vi "GUI_HTU_Camera_presets.vi"() -> ()   [LabVIEW 2013]
uses:
  Shared/GUI_Template/GUI_master/tcp_new_data_event.ctl
  Shared/GUI_Template/GUI_master/tcp new data cluster.ctl
panel:
  in  "OapIn2AA":dbl=0.01
  in  "OapIn1AA":dbl=0.001
  in  "expanderIn2AA":dbl=0.0001
  in  "compInAA":dbl=0.001
  in  "BeamlineOutAA":dbl=0.0001
  in  "BeamlineInAA":dbl=0.0001
  in  "tubeInAA":dbl=0.0001
  in  "DMSurfaceAA":dbl=0.01
  in  "BcaveInAA":dbl=0.0001
  in  "group4":bool caption="Blank Button"
  in  "group3":bool caption="Blank Button"
  in  "amp2inputAA 2":dbl=0.001
  in  "amp3inputAA 2":dbl=0.001
  in  "amp4inputAA 2":dbl=0.001
  in  "amp4outputAA 2":dbl=0.001
  in  "BcaveInAA 2":dbl=0.002
  in  "DMSurfaceAA 2":dbl=0.8
  in  "tubeInAA 2":dbl=0.02
  in  "BeamlineInAA 2":dbl=0.01
  in  "BeamlineOutAA 2":dbl=0.08
  in  "compInAA 2":dbl=0.07
  in  "expanderIn2AA 2":dbl=0.005
  in  "OapIn1AA 2":dbl=0.2
  in  "OapIn2AA 2":dbl=0.8
  in  "amp4outputAA":dbl=0.9
  in  "amp4inputAA":dbl=0.7
  in  "amp3inputAA":dbl=0.5
  in  "group2":bool caption="Blank Button"
  in  "amp2inputAA":dbl=0.002
  in  "exposure::18":dbl caption="TubeIn" min=50.0 max=500000.0
  in  "exposure::17":dbl caption="OapIn2" min=0.0001 max=1.0
  in  "exposure::16":dbl caption="OapIn1" min=0.0001 max=1.0
  in  "exposure::15":dbl caption="ModeImager" min=2e-05 max=1.0
  in  "exposure::14":dbl caption="GratingMode" min=1e-05 max=1.0
  in  "exposure::13":dbl caption="GhostPulsed" min=0.0 max=1.0
  in  "exposure::12":dbl caption="ExpanderIn2" min=3e-05 max=1.0
  in  "exposure::11":dbl caption="ExpanderIn1Pulsed" min=1e-06 max=1.0
  in  "exposure::10":dbl caption="ExapnderIn1" min=3e-05 max=1.0
  in  "exposure::9":dbl caption="DMSurface" min=20.0 max=1000000.0
  in  "exposure::8":dbl caption="compIn" min=2e-05 max=4.0
  in  "exposure::7":dbl caption="beamlineOUt" min=0.0001 max=1.0
  in  "exposure::6":dbl caption="beamlineIn" min=0.0001 max=1.0
  in  "exposure::5":dbl caption="bcavein" min=10.0 max=1000000.0
  in  "exposure::4":dbl caption="amp4Outpur" min=-25.0 max=25.0
  in  "exposure::3":dbl caption="Amp4input" min=0.0001 max=1.0
  in  "exposure::2":dbl caption="amp3input" min=0.0001 max=1.0
  in  "ms exposure":dbl=0.001
  in  "group1":bool caption="Blank Button"
  in  "GUIdevice 18":string="UC_TubeIn"
  in  "GUIdevice 17":string="UC_OAPin2"
  in  "GUIdevice 16":string="UC_OAPin1"
  in  "GUIdevice 15":string="UC_ModeImager"
  in  "GUIdevice 14":string="UC_GratingMode"
  in  "GUIdevice 13":string="UC_Ghost_Pulsed"
  in  "GUIdevice 12":string="UC_ExpanderIn2"
  in  "GUIdevice 11":string="UC_ExpanderIn1_Pulsed"
  in  "GUIdevice 10":string="UC_ExpanderIn1"
  in  "GUIdevice 9":string="UC_DMSurface"
  in  "GUIdevice 8":string="UC_CompIn"
  in  "exposure::1":dbl caption="amp2Input" min=0.0001 max=1.0
  in  "GUIdevice 6":string="UC_Beamline_In"
  in  "GUIdevice 5":string="UC_BCaveIn"
  out "error IO 2":errorcluster
  out "tcp data event":T1
  in  "UDP error message":string
  in  "GUIdevice 7":string="UC_Beamline_Out"
  in  "GUIdevice 2":string="UC_Amp3_IR_input"
  in  "GUIdevice 4":string="UC_Amp4_output"
  in  "GUIdevice 1":string="UC_Amp2_IR_input"
  in  "GUIdevice 3":string="UC_Amp4_IR_input"
  in  "stop":bool
  # "Camera exposure controls"
  # "Direct control"
  # "Energy"
  # "CAP"
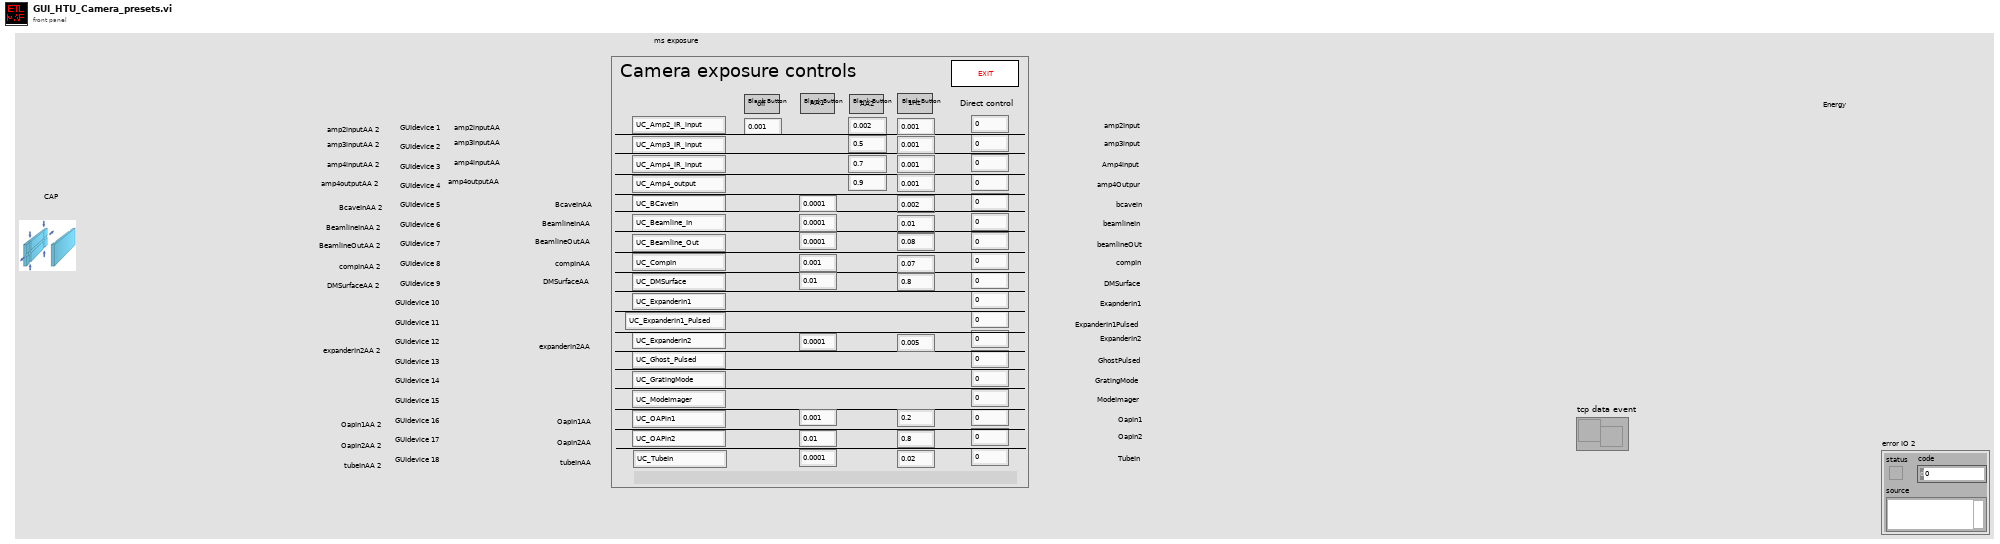
[diagram p1: front panel]
types:
  T1 = typedef "tcp_new_data_event.ctl" = refnum<user-event>
  T2 = typedef "tcp new data cluster.ctl" = cluster{"EventEnum":enum16{"new data", "connection status update"}, "Device name":string}
  T3 = enum32{"invalid app kind", "Development System", "Run Time System", "Student Edition", "Embedded LabVIEW", "Evaluation", "Custom"}
  T4 = enum32{"Invalid", "Standard", "Closed", "Hidden", "Minimized", "Maximized"}
  T5 = cluster{"Core":cluster{"Current VI Reference":refnum<vi>, "Close Panel on Exit?":bool}, "Heater timing offset":dbl, "Discharge timing offset":dbl, "Jet trigger":bool, "Tik1":u32, "Tik2":u32, "Fire Continues Allowed":bool, "Jet enable":bool, "Wedge enable":bool, "Phosphor enable":bool, "last chart update tck":i32}
  T6 = cluster{"Current VI Reference":refnum<vi>, "Close Panel on Exit?":bool}
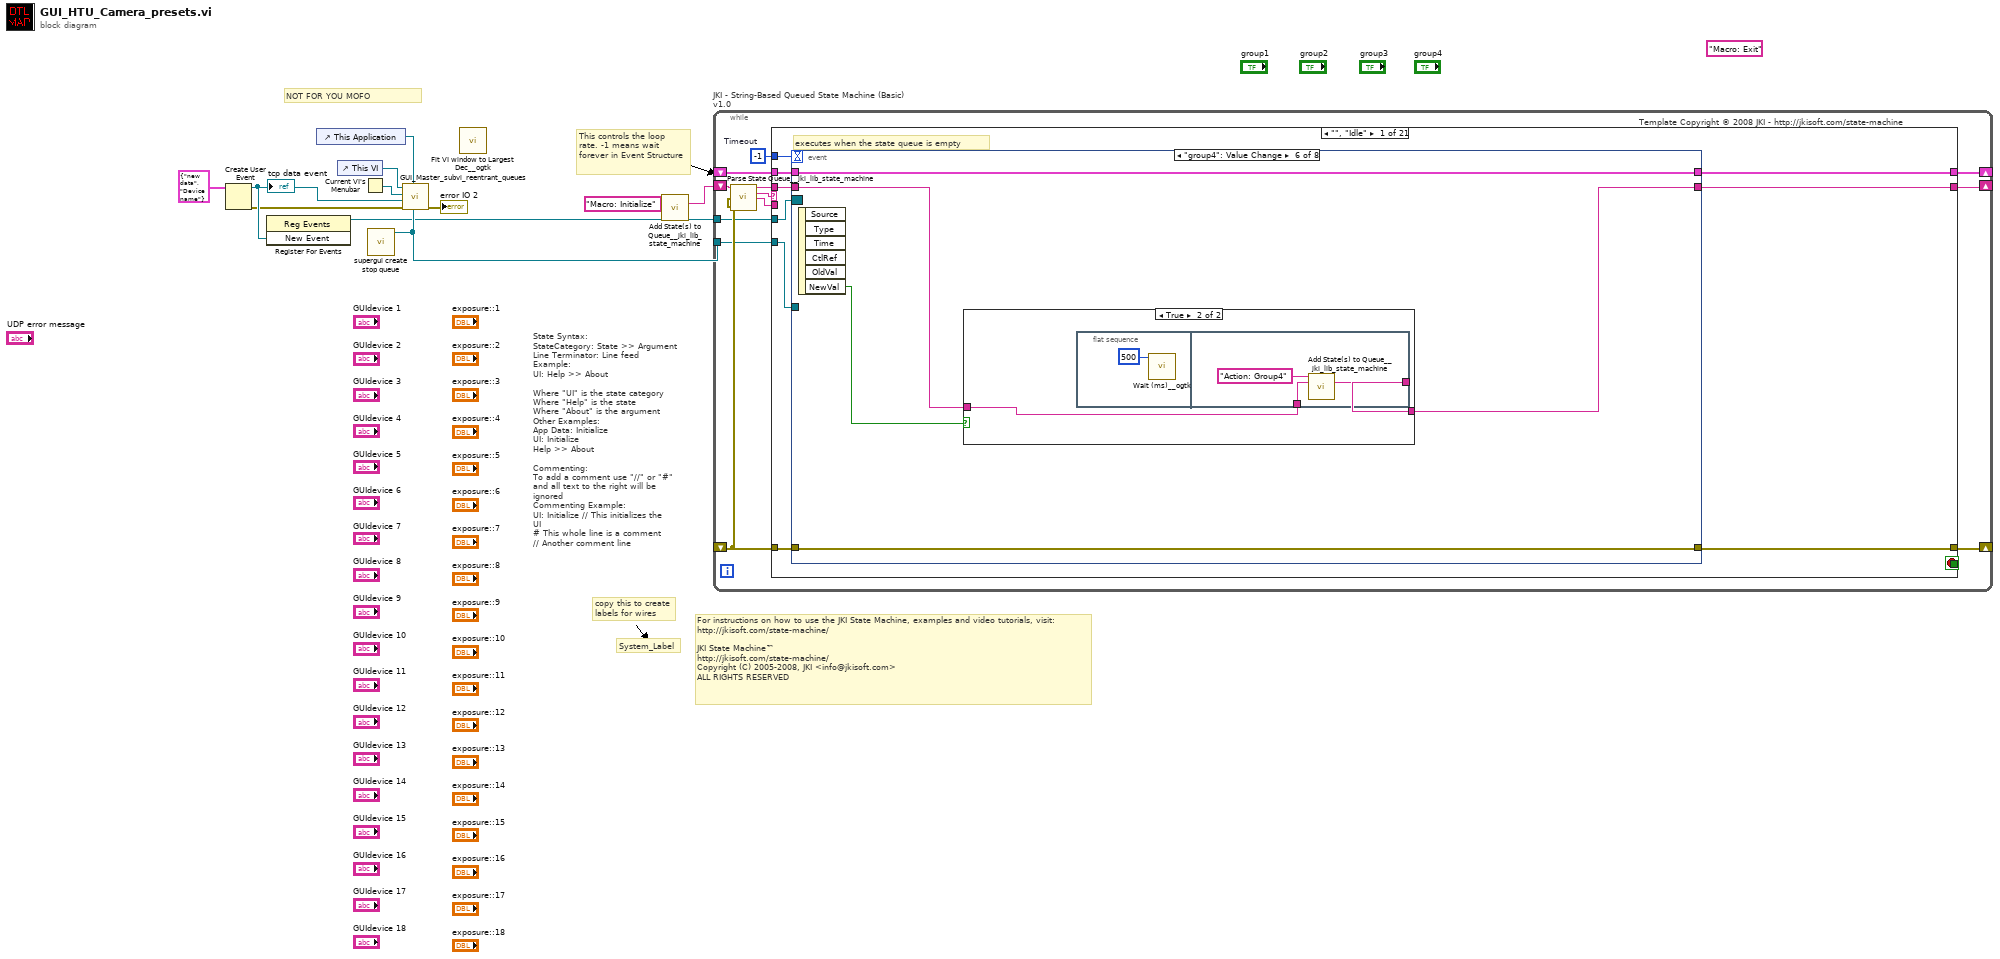
[diagram p0: block diagram]
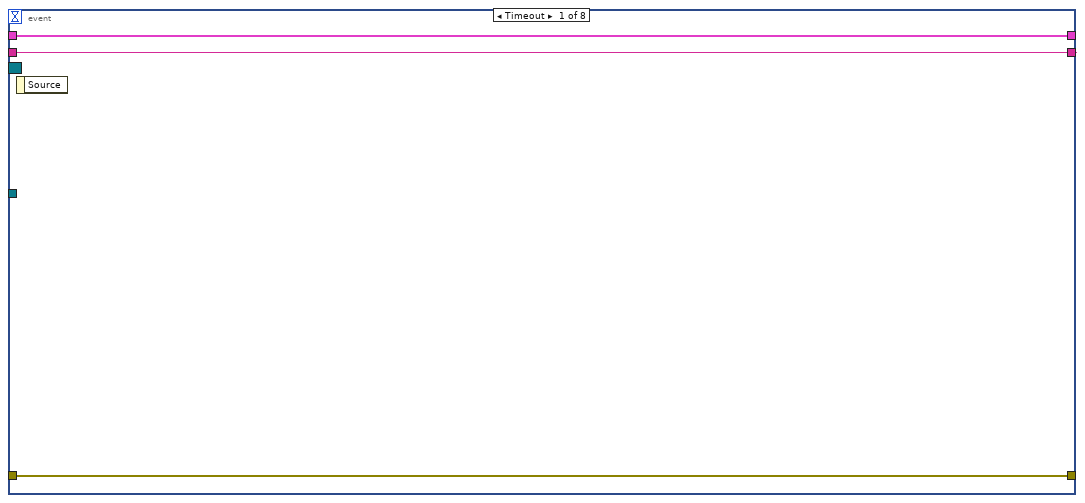
[diagram p2: hidden frame]
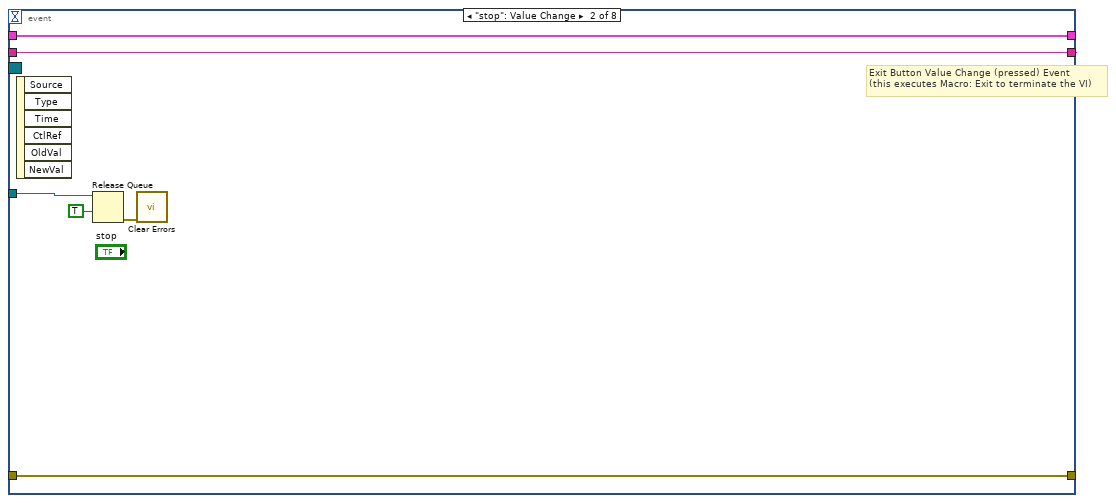
[diagram p3: hidden frame]
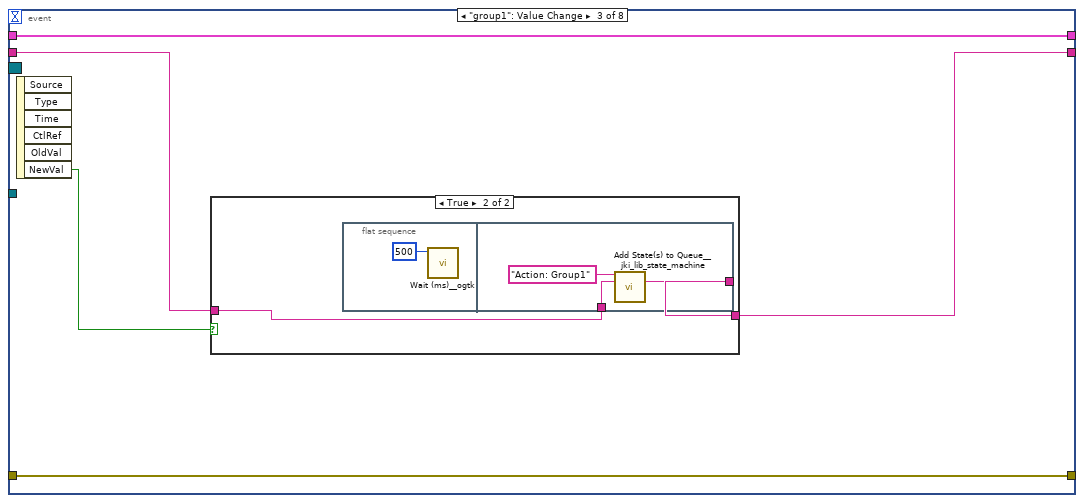
[diagram p4: hidden frame]
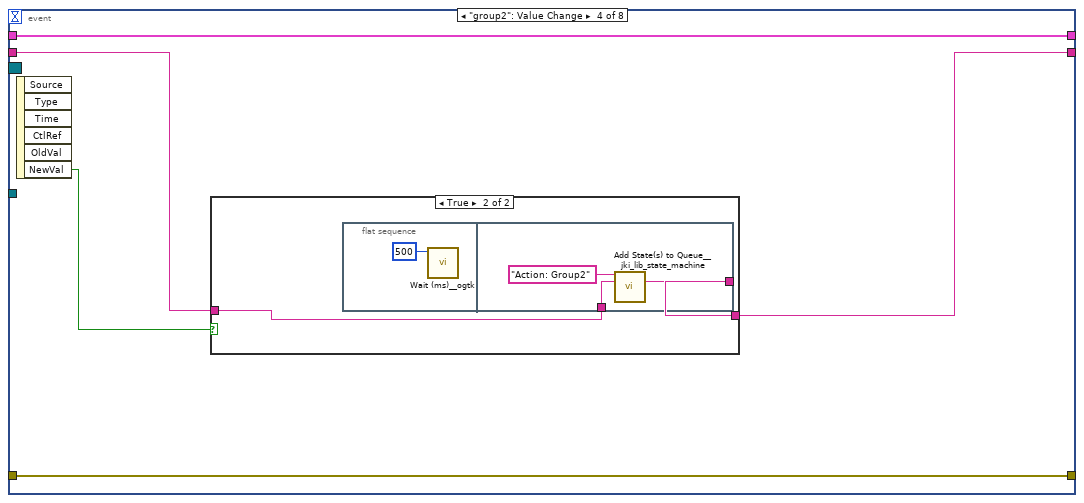
[diagram p6: hidden frame]
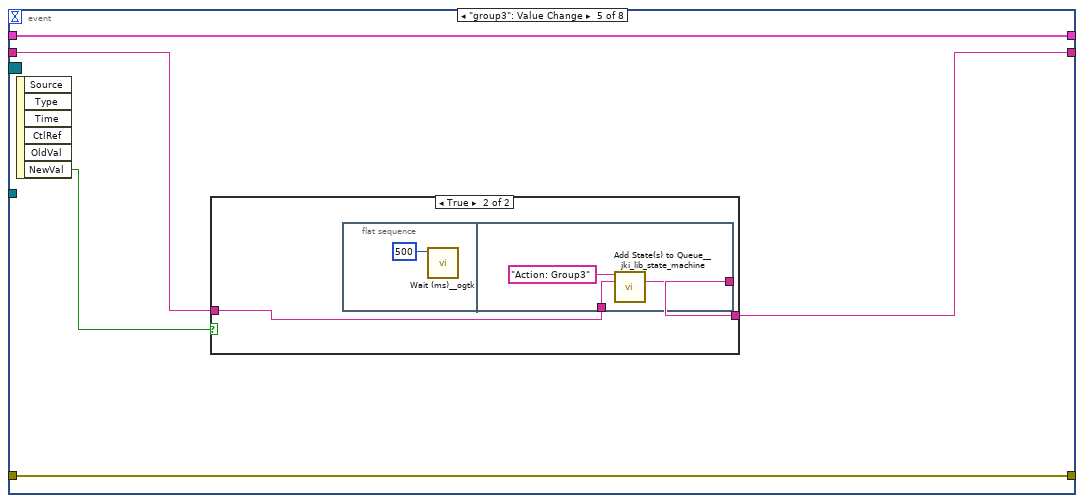
[diagram p8: hidden frame]
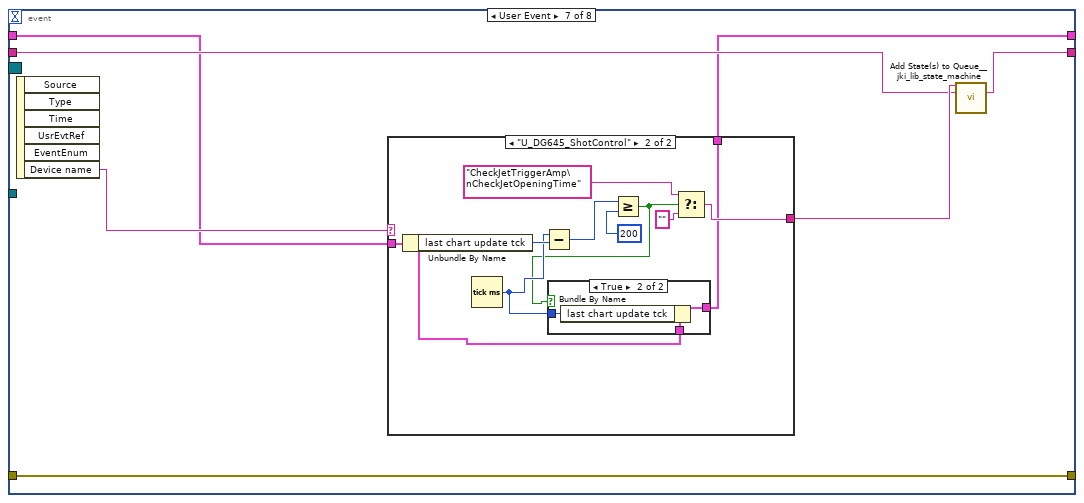
[diagram p11: hidden frame]
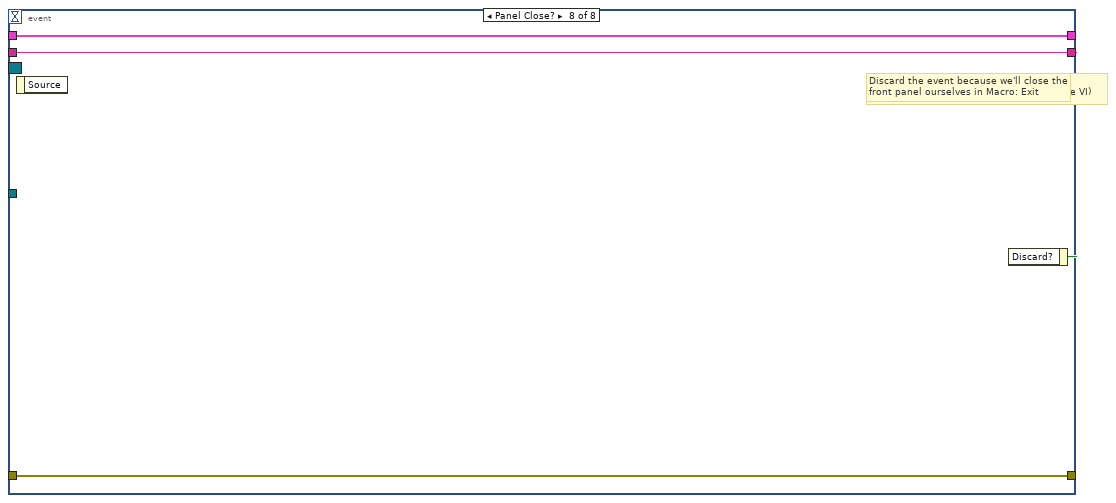
[diagram p14: hidden frame]
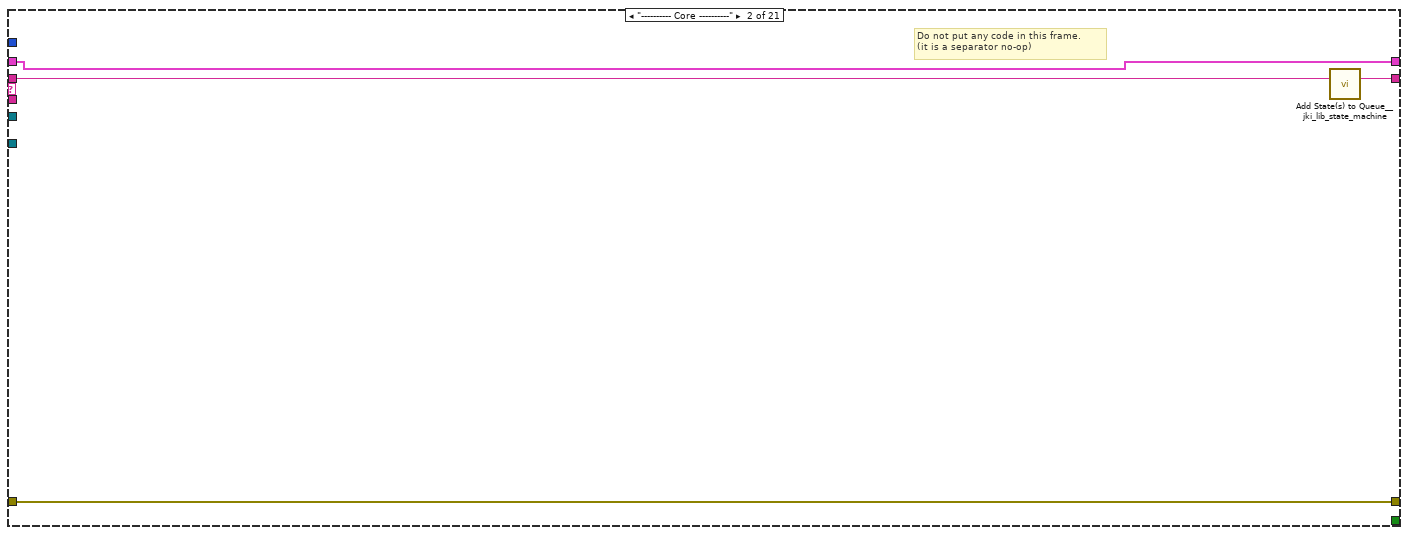
[diagram p15: hidden frame]
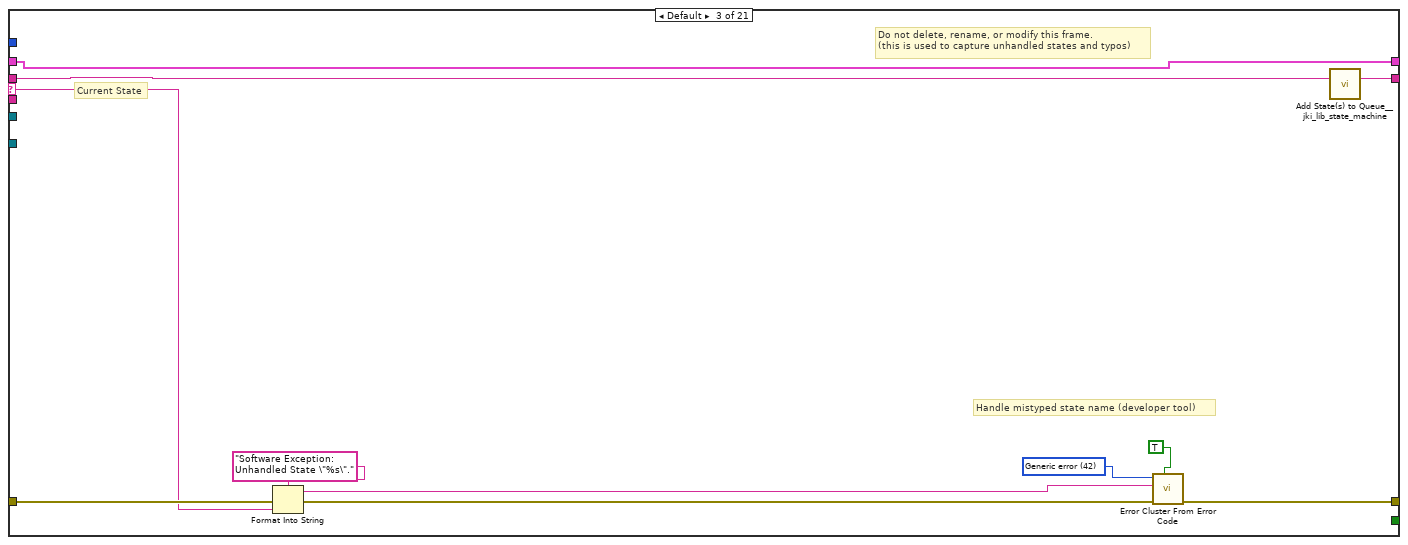
[diagram p16: hidden frame]
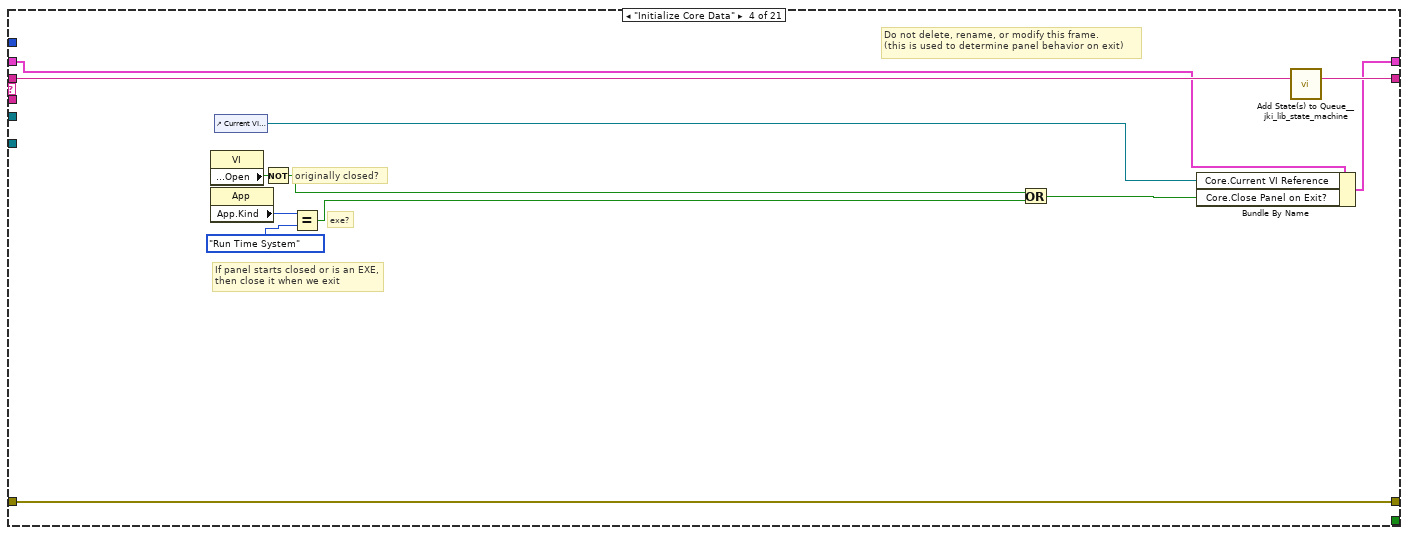
[diagram p17: hidden frame]
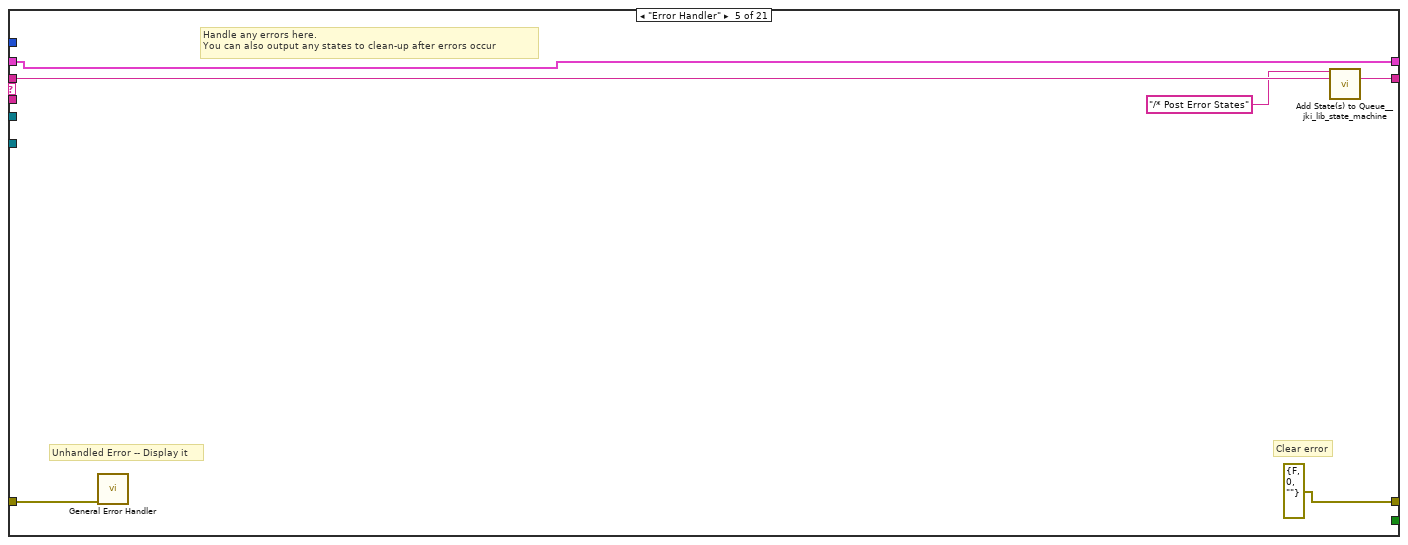
[diagram p18: hidden frame]
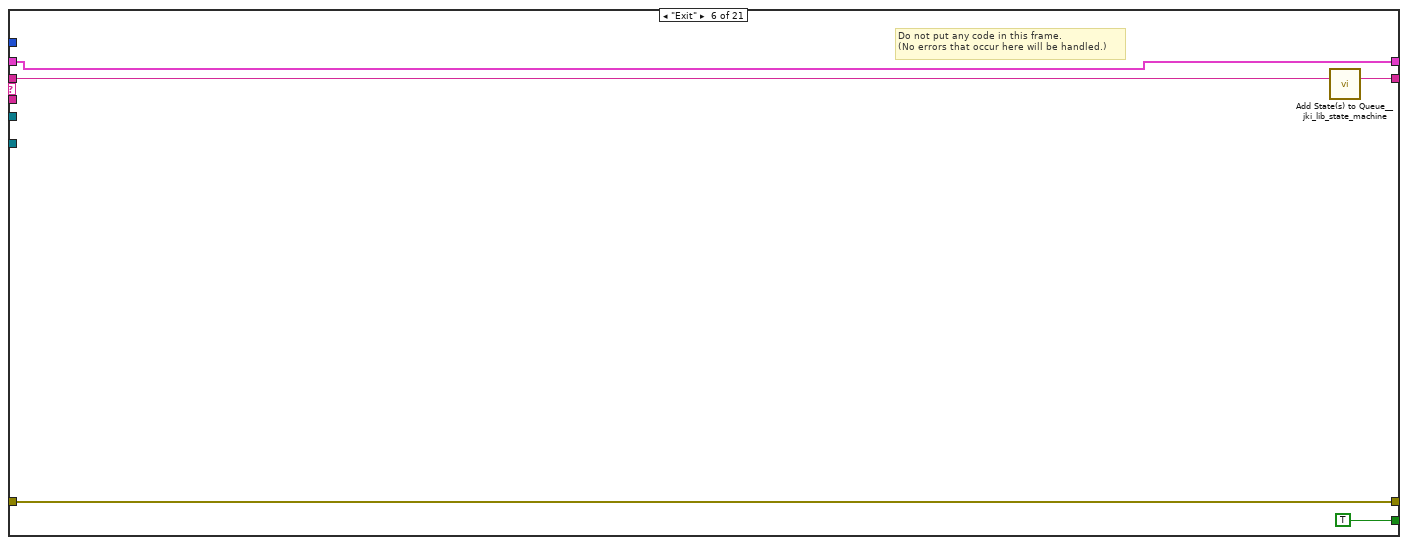
[diagram p19: hidden frame]
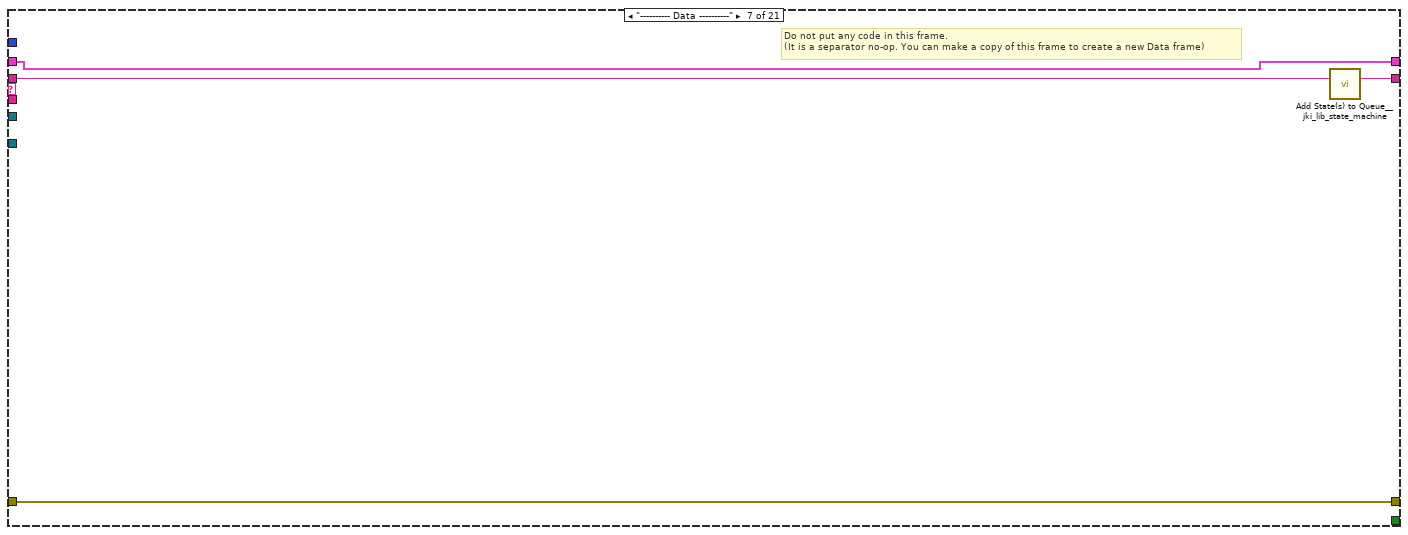
[diagram p20: hidden frame]
diagram:
  (unwired) "Macro: Exit"
  # "For instructions on how to use the JKI State Machine, examples and video tutorials, visit:\nhttp://jkisoft.com/state-machine/\n\nJKI State Machine™\nhttp://jkisoft.com/state-machine/\nCopyright (C) 2005-2008, JKI <info@jkisoft.com>\nALL RIGHTS RESERVED"
  # "State Syntax:\nStateCategory: State >> Argument\nLine Terminator: Line feed\nExample:\nUI: Help >> About\n\nWhere \"UI\" is the state category\nWhere \"Help\" is the state\nWhere \"About\" is the argument\nOther Examples:\nApp Data: Initialize\nUI: Initialize\nHelp >> About\n\nCommenting:\nTo add a comment use \"//\" or \"#\" and all text to the right will be ignored\nCommenting Example:\nUI: Initialize // This initializes the UI\n# This whole line is a comment\n// Another comment line"
  # "copy this to create labels for wires"
  # "This controls the loop rate. -1 means wait forever in Event Structure"
  # "System_Label"
  # "NOT FOR YOU MOFO"
  n1 = Create User Event(user event datatype=T2 {"EventEnum"=enum."new data", "Device name"="Device name"} ("New Event")) -> (user event=w10:refnum<user-event>, error out=w9:errorcluster)  [unwired: 1 in]
  "tcp data event" <- w10
  n2 = register-events(w10) -> (reference out=w1:refnum<event-registration>)  [unwired: 2 in, 1 out]
  n3 = control-ref of="This Application"() -> (w11:refnum<vi>)
  n4 = control-ref of="This VI"() -> (w5:refnum<vi>)
  n5 = Current VI's Menubar() -> (w7:refnum<k9>)
  n6 = call "supergui create stop queue.vi"() -> ("STOP Queue out"=w2:refnum<queue>)  [unwired: 11 in]
  n7 = call "GUI_Master_subvi_reentrant_queues.vi"("STOP Queue in"=w2, "This Application"=w11, "error in (no error)"=w9, "tcp data event"=w10, "Caller menu reference"=w7, "Caller VI ref"=w5) -> ("error out"=→"error IO 2":errorcluster)  [unwired: 5 in]
  n8 = call <userlib>:"Fit VI window to Largest Dec__ogtk.vi"() -> ()  [unwired: 6 in, 2 out]
  n9 = call <vilib>:"Add State(s) to Queue__jki_lib_state_machine.vi"("State(s) in (\"\")"="Macro: Initialize") -> ("States Out"=w3:string)  [unwired: 14 in]
  n10 = while "JKI - String-Based Queued State Machine (Basic) v1.0" {
    shift-right: [w17] -> _
    shift-left: _ -> [w16]
    shift-right: [w20] -> _
    shift-left: _ -> [w14]
    shift-right: [w19] -> _
    shift-left: w3 -> [w21]
    tunnel: w1 -> [w13]
    tunnel: w2 -> [w12]
    stop <- w18 stop-if-true
    w15 = -1  # Timeout
    # "Template Copyright © 2008 JKI - http://jkisoft.com/state-machine"
    n11 = call <vilib>:"Parse State Queue__jki_lib_state_machine.vi"("State Queue"=w21, "Error In (no error)"=w14) -> ("Remaining States"=w23:string, "Current State"=w24:string, "Arguments"=w22:string)  [unwired: 11 in]
    n12 = case shown="\"\", \"Idle\"" w24 {
      selector: w24 -> [_ _ w126 _ _ _ _ _ _ _ _ _ _ _ _ _ _ _ _ _ _]
      tunnel: w23 -> [w33 w125 w130 w148 w154 w159 w163 w178 w184 w188 w192 w198 w209 w235 w240 w250 w254 w279 w292 w327 w353]
      tunnel: w22 -> [_ _ _ _ _ _ _ _ _ _ _ w193 w203 _ _ _ _ _ _ _ _]
      tunnel: w16 -> [w31 w122 w128 w139 w151 w157 w160 _ w179 w185 w190 w196 w205 w232 w237 w247 w251 w277 w290 w325 w351]
      tunnel: [w30 w123 w132 w145 errorcluster {"status"=FALSE, "code"=0, "source"=""} ("error out") w156 w161 w175 w180 w186 w189 w194 w206 w233 w238 w248 w252 w255 w283 w311 w328] -> w20
      tunnel: w14 -> [w29 w123 w131 w145 w150 w156 w161 w175 w181 w186 w189 w195 w207 w233 w238 w248 w252 w276 w289 w324 w329]
      tunnel: [w32 w124 w129 w147 w153 w158 w162 w177 w183 w187 w191 w197 w208 w234 w239 w249 w253 w278 w291 w326 w352] -> w19
      tunnel: [_ _ _ _ _ TRUE _ _ _ _ _ _ _ _ _ _ _ _ _ _ _] -> w18
      tunnel: [w25 w122 w128 w146 w151 w157 w160 w176 w179 w185 w190 w196 w205 w232 w237 w247 w251 w277 w290 w325 w351] -> w17
      tunnel: w15 -> [w28 _ _ _ _ _ _ _ _ _ _ _ _ _ _ _ _ _ _ _ _]
      tunnel: w13 -> [w27 _ _ _ _ _ _ _ _ _ _ _ _ _ _ _ _ _ _ _ _]
      tunnel: w12 -> [w26 _ _ _ _ _ _ _ _ _ _ _ _ _ _ _ _ _ _ _ _]
      frame "", "Idle" {
        # "executes when the state queue is empty"
        n13 = event shown="[5] \"group4\": Value Change" {
          selector: w27 -> [_ _ _ _ _ _ _ _]
          dyn-events: _ -> [_ _ _ _ _ _ _ _]
          timeout: w28 -> [_ _ _ _ _ _ _ _]
          tunnel: w33 -> [w37 w45 w46 w58 w70 w82 w97 w121]
          tunnel: [w36 w44 w47 w59 w71 w83 w96 w120] -> w32
          tunnel: w31 -> [w34 w42 w49 w61 w73 w85 w95 w118]
          tunnel: [w35 w43 w50 w62 w74 w86 w100 w119] -> w30
          tunnel: w29 -> [w35 w43 w50 w62 w74 w86 w100 w119]
          tunnel: [w34 w42 w49 w61 w73 w85 w94 w118] -> w25
          tunnel: w26 -> [_ w39 _ _ _ _ _ _]
          event Timeout {
            n14 = event-data() -> ()  [unwired: 1 in, 1 out]
            n15 = call <vilib>:"Add State(s) to Queue__jki_lib_state_machine.vi"("State(s) in (\"\")"=w37) -> ("States Out"=w36:string)  [unwired: 14 in]
          }
          event "stop": Value Change {
            # "Exit Button Value Change (pressed) Event\n(this executes Macro: Exit to terminate the VI)"
            n16 = event-data() -> ()  [unwired: 1 in, 6 out]
            n17 = Release Queue(queue=w39, force destroy? (F)=TRUE) -> (error out=w40:errorcluster)  [unwired: 1 in, 2 out]
            n18 = call <vilib>:"Clear Errors.vi"("error in (no error)"=w40) -> ()  [unwired: 6 in, 1 out]
            n19 = call <vilib>:"Add State(s) to Queue__jki_lib_state_machine.vi"("State(s) in Front (\"\")"="Macro: Exit", "State(s) in (\"\")"=w45) -> ("States Out"=w44:string)  [unwired: 13 in]
          }
          event "group1": Value Change {
            n20 = event-data() -> ("NewVal"=w48:bool)  [unwired: 1 in, 5 out]
            n21 = case shown="True" w48 {
              tunnel: [w51 w53] -> w47
              tunnel: w46 -> [w51 w52]
              frame False {
              }
              frame True {
                n22 = flat-sequence {
                  tunnel: [w56] -> w53
                  tunnel: w52 -> [w55]
                  frame #0 {
                    n23 = call <userlib>:"Wait (ms)__ogtk.vi"("milliseconds to wait"=u32 500) -> ()  [unwired: 9 in, 2 out]
                  }
                  frame #1 {
                    n24 = call <vilib>:"Add State(s) to Queue__jki_lib_state_machine.vi"("State(s) in Front (\"\")"="Action: Group1" ("State(s) in Front (\"\")"), "State(s) in (\"\")"=w55) -> ("States Out"=w56:string)  [unwired: 13 in]
                  }
                }
              }
            }
          }
          event "group2": Value Change {
            n25 = event-data() -> ("NewVal"=w60:bool)  [unwired: 1 in, 5 out]
            n26 = case shown="True" w60 {
              tunnel: [w63 w65] -> w59
              tunnel: w58 -> [w63 w64]
              frame False {
              }
              frame True {
                n27 = flat-sequence {
                  tunnel: [w68] -> w65
                  tunnel: w64 -> [w67]
                  frame #0 {
                    n28 = call <userlib>:"Wait (ms)__ogtk.vi"("milliseconds to wait"=u32 500) -> ()  [unwired: 9 in, 2 out]
                  }
                  frame #1 {
                    n29 = call <vilib>:"Add State(s) to Queue__jki_lib_state_machine.vi"("State(s) in Front (\"\")"="Action: Group2" ("State(s) in Front (\"\")"), "State(s) in (\"\")"=w67) -> ("States Out"=w68:string)  [unwired: 13 in]
                  }
                }
              }
            }
          }
          event "group3": Value Change {
            n30 = event-data() -> ("NewVal"=w72:bool)  [unwired: 1 in, 5 out]
            n31 = case shown="True" w72 {
              tunnel: [w75 w77] -> w71
              tunnel: w70 -> [w75 w76]
              frame False {
              }
              frame True {
                n32 = flat-sequence {
                  tunnel: [w80] -> w77
                  tunnel: w76 -> [w79]
                  frame #0 {
                    n33 = call <userlib>:"Wait (ms)__ogtk.vi"("milliseconds to wait"=u32 500) -> ()  [unwired: 9 in, 2 out]
                  }
                  frame #1 {
                    n34 = call <vilib>:"Add State(s) to Queue__jki_lib_state_machine.vi"("State(s) in Front (\"\")"="Action: Group3" ("State(s) in Front (\"\")"), "State(s) in (\"\")"=w79) -> ("States Out"=w80:string)  [unwired: 13 in]
                  }
                }
              }
            }
          }
          event "group4": Value Change {
            n35 = event-data() -> ("NewVal"=w84:bool)  [unwired: 1 in, 5 out]
            n36 = case shown="True" w84 {
              tunnel: [w87 w89] -> w83
              tunnel: w82 -> [w87 w88]
              frame False {
              }
              frame True {
                n37 = flat-sequence {
                  tunnel: [w92] -> w89
                  tunnel: w88 -> [w91]
                  frame #0 {
                    n38 = call <userlib>:"Wait (ms)__ogtk.vi"("milliseconds to wait"=u32 500) -> ()  [unwired: 9 in, 2 out]
                  }
                  frame #1 {
                    n39 = call <vilib>:"Add State(s) to Queue__jki_lib_state_machine.vi"("State(s) in Front (\"\")"="Action: Group4" ("State(s) in Front (\"\")"), "State(s) in (\"\")"=w91) -> ("States Out"=w92:string)  [unwired: 13 in]
                  }
                }
              }
            }
          }
          event User Event {
            n40 = event-data() -> ("Device name"=w99:string)  [unwired: 1 in, 5 out]
            n41 = case shown="\"U_DG645_ShotControl\"" w99 {
              tunnel: [_ w105] -> w98
              tunnel: w95 -> [w101 w103]
              tunnel: [w101 w102] -> w94
              frame "False", Default {
              }
              frame "U_DG645_ShotControl" {
                n42 = Unbundle By Name(w103) -> ("last chart update tck"=w111:i32)
                n43 = Tick Count (ms)() -> (millisecond timer value=w107:u32)
                n44 = Subtract(x=w107, y=w111) -> (x-y=w110:u32)
                n45 = Greater Or Equal?(x=w110, y=u32 200 ("x")) -> (x >= y?=w106:bool)
                n46 = case shown="True" w106 {
                  tunnel: [w112 w115] -> w102
                  tunnel: w103 -> [w112 w114]
                  tunnel: w107 -> [_ w113]
                  frame False {
                  }
                  frame True {
                    n47 = Bundle By Name(cluster=w114, "last chart update tck"=w113) -> (w115:T5)
                  }
                }
                n48 = Select(t="CheckJetTriggerAmp\nCheckJetOpeningTime", s=w106, f="") -> (s? t:f=w105:string)
              }
            }
            n49 = call <vilib>:"Add State(s) to Queue__jki_lib_state_machine.vi"("State(s) in Front (\"\")"=w98, "State(s) in (\"\")"=w97) -> ("States Out"=w96:string)  [unwired: 13 in]
          }
          event Panel Close? {
            # "Discard the event because we'll close the front panel ourselves in Macro: Exit"
            # "Close Panel button (pressed) Event\n(this executes Macro: Exit to terminate the VI)"
            n50 = event-data() -> ()  [unwired: 1 in, 1 out]
            n51 = event-data("Discard?"=TRUE) -> ()  [unwired: 1 in, 1 out]
            n52 = call <vilib>:"Add State(s) to Queue__jki_lib_state_machine.vi"("State(s) in Front (\"\")"="Macro: Exit", "State(s) in (\"\")"=w121) -> ("States Out"=w120:string)  [unwired: 13 in]
          }
        }
      }
      frame "---------- Core ----------" {
        # "Do not put any code in this frame.\n(it is a separator no-op)"
        n53 = call <vilib>:"Add State(s) to Queue__jki_lib_state_machine.vi"("State(s) in (\"\")"=w125) -> ("States Out"=w124:string)  [unwired: 14 in]
      }
      frame Default {
        w135 = 42 items=["No error", "Argument error", "Memory is full", "Out of zone", "End of file", "File already open", "Generic file I/O error", "File not found", "File permission error", "Disk is full", "Duplicate path", "Too many files open", "System feature not enabled", "Resource file not found", "Cannot add resource", "Resource not found", "Image not found", "Image memory error", "Pen does not exist", "Config type invalid", "Config token not found", "Config parse error", "Config memory error", "Bad external code format", "Bad external code offset", "External code not present", "Null window", "Destroy window error", "Null menu", "Print aborted", "Bad print record", "Print driver error", "Windows error during printing", "Memory error during printing", "Print dialog error", "Generic print error", "Invalid device refnum", "Device not found", "Device parameter error", "Device unit error", "Cannot open device", "Device call aborted", "Generic error", "Cancelled by user", "Object ID too low", "Object ID too high", "Object not in heap", "Unknown heap", "Unknown object (invalid DefProc)", "Unknown object (DefProc not in table)", "Message out of range", "Invalid (null) method", "Unknown message", "Manager call not supported", "Bad address", "Network operation in progress", "Network operation timed out", "Connection is busy", "Network attribute not supported", "Network error", "Address in use", "System out of memory", "Connection aborted", "Connection refused", "Not connected", "Already connected", "Connection closed", "Initialization error (interapplication manager)", "Bad occurrence", "Wait on unbound occurrence handler", "Occurrence queue overflow", "Datalog type conflict", "Unused", "Unrecognized type (interapplication manager)", "Memory corrupt", "Failed to make temporary DLL", "Old CIN version", "Drag socket not found", "Failed to load drop-object", "Failed to register OLE object", "Failed to release OLE object", "Format specifier type mismatch", "Unknown format specifier", "Too few format specifiers", "Too many format specifiers", "Scan failed", "Newer CIN version", "Error converting to variant", "Runtime menu error", "Password tampered", "Variant attribute not found", "Incompatible variant data type", "Event data is not available", "Event Store is not present", "Occurrence is not found", "Event Queue is not created", "Event info is not available", "Refnum passed is NULL", "Error retrieving Class GUID", "Error retrieving CoClass GUID", "Error retrieving TypeLib GUID.", "Bad built application magic bytes.", "Specific driver is different from the specific driver associated with the Logical Name.", "There is no session opened to the class driver.", "Max Error", "MAX - Error with config objects", "MAX - Error loading configuration", "MAX - Group not supported"]
        # "Current State"
        # "Do not delete, rename, or modify this frame.\n(this is used to capture unhandled states and typos)"
        # "Handle mistyped state name (developer tool)"
        n54 = Format Into String(format string="Software Exception: Unhandled State \"%s\"." ("message"), error in=w131, w126) -> (resulting string=w134:string, error out=w133:errorcluster)  [unwired: 1 in]
        n55 = call <vilib>:"Error Cluster From Error Code.vi"("show call chain? (False)"=TRUE, "error in (no error)"=w133, "error message (\"\")"=w134, "error code (0)"=w135) -> ("error out"=w132:errorcluster)  [unwired: 5 in]
        n56 = call <vilib>:"Add State(s) to Queue__jki_lib_state_machine.vi"("State(s) in (\"\")"=w130) -> ("States Out"=w129:string)  [unwired: 14 in]
      }
      frame "Initialize Core Data" {
        # "Do not delete, rename, or modify this frame.\n(this is used to determine panel behavior on exit)"
        # "originally closed?"
        # "exe?"
        # "If panel starts closed or is an EXE, then close it when we exit"
        n57 = property class="VI"() -> ("Front Panel.Open"=w144:bool)  [unwired: 2 in, 2 out]
        n58 = property class="App"() -> ("App.Kind"=w143:T3)  [unwired: 2 in, 2 out]
        n59 = control-ref of="Current VI Reference"() -> (w137:refnum<vi>)
        n60 = Not(x=w144) -> (.not. x?=w141:bool)
        n61 = Equal?(x=w143, y=T3."Run Time System" ("Application:Kind")) -> (x = y?=w140:bool)
        n62 = Or(x=w141, y=w140) -> (x .or. y?=w138:bool)
        n63 = Bundle By Name(cluster=w139, "Core.Current VI Reference"=w137, "Core.Close Panel on Exit?"=w138) -> (w146:T5)
        n64 = call <vilib>:"Add State(s) to Queue__jki_lib_state_machine.vi"("State(s) in (\"\")"=w148) -> ("States Out"=w147:string)  [unwired: 14 in]
      }
      frame "Error Handler" {
        # "Unhandled Error -- Display it"
        # "Handle any errors here.\nYou can also output any states to clean-up after errors occur"
        # "Clear error"
        n65 = call <vilib>:"General Error Handler.vi"("error in (no error)"=w150) -> ()  [unwired: 10 in, 5 out]
        n66 = call <vilib>:"Add State(s) to Queue__jki_lib_state_machine.vi"("State(s) in Front (\"\")"="/* Post Error States", "State(s) in (\"\")"=w154) -> ("States Out"=w153:string)  [unwired: 13 in]
      }
      frame "Exit" {
        # "Do not put any code in this frame.\n(No errors that occur here will be handled.)"
        n67 = call <vilib>:"Add State(s) to Queue__jki_lib_state_machine.vi"("State(s) in (\"\")"=w159) -> ("States Out"=w158:string)  [unwired: 14 in]
      }
      frame "---------- Data ----------" {
        # "Do not put any code in this frame.\n(It is a separator no-op. You can make a copy of this frame to create a new Data frame)"
        n68 = call <vilib>:"Add State(s) to Queue__jki_lib_state_machine.vi"("State(s) in (\"\")"=w163) -> ("States Out"=w162:string)  [unwired: 14 in]
      }
      frame "Data: Initialize" {
        w164 = 0  # last chart update tck
        w165 = FALSE  # Phosphor enable
        w166 = FALSE  # Wedge enable
        w167 = FALSE  # Jet enable
        w168 = FALSE  # Fire Continues Allowed
        w170 = u32 0  # Tik1
        w169 = u32 0  # Tik2
        w171 = FALSE  # Jet trigger
        w172 = 0.0  # Discharge timing offset
        w173 = 0.0  # Heater timing offset
        w174 = T6 {"Current VI Reference"=refnum, "Close Panel on Exit?"=FALSE}  # Core
        # "do not delete - used by framework"
        # "Expand Bundle to add new data elements to shift register data."
        # "Add new data here."
        # "Data names and types of shift register data are defined by this bundle."
        # "Initialize the shift-register data, here.\n(data names are defined by what you wire into the bundle function)"
        n69 = Bundle("Core"=w174, "Heater timing offset"=w173, "Discharge timing offset"=w172, "Jet trigger"=w171, "Tik1"=w170, "Tik2"=w169, "Fire Continues Allowed"=w168, "Jet enable"=w167, "Wedge enable"=w166, "Phosphor enable"=w165, "last chart update tck"=w164) -> (w176:T5)  [unwired: 1 in]
        n70 = call <vilib>:"Add State(s) to Queue__jki_lib_state_machine.vi"("State(s) in (\"\")"=w178) -> ("States Out"=w177:string)  [unwired: 14 in]
      }
      frame "Data: Cleanup" {
        # "Cleanup any data and references, here.\n(this is called automatically, by the Macro: Exit)"
        n71 = Unbundle By Name(w179) -> ("Core.Current VI Reference"=w182:refnum<vi>)
        n72 = Close Reference(reference=w182, error in (no error)=w181) -> (error out=w180:errorcluster)
        n73 = call <vilib>:"Add State(s) to Queue__jki_lib_state_machine.vi"("State(s) in (\"\")"=w184) -> ("States Out"=w183:string)  [unwired: 14 in]
      }
      frame "---------- UI ----------" {
        # "Do not put any code in this frame.\n(It is a separator no-op. You can make a copy of this frame to create a new UI frame)"
        n74 = call <vilib>:"Add State(s) to Queue__jki_lib_state_machine.vi"("State(s) in (\"\")"=w188) -> ("States Out"=w187:string)  [unwired: 14 in]
      }
      frame "UI: Initialize" {
        # "Initialize the User Interface, here.\n(this is called automatically, by the Macro: Init)"
        n75 = call <vilib>:"Add State(s) to Queue__jki_lib_state_machine.vi"("State(s) in (\"\")"=w192) -> ("States Out"=w191:string)  [unwired: 14 in]
      }
      frame "UI: Cursor Set" {
        # "Argument"
        # "Set and Unset Cursor Busy.\n(Usage: \"UI: Cursor Set >> Busy|Idle\")"
        n76 = case shown="\"Idle\", Default" w193 {
          tunnel: w195 -> [w200 w202]
          tunnel: [w199 w201] -> w194
          frame "Idle", Default {
            n77 = call <vilib>:"Unset Busy.vi"("error in (no error)"=w200) -> ("error out"=w199:errorcluster)  [unwired: 10 in]
          }
          frame "Busy" {
            n78 = call <vilib>:"Set Busy.vi"("error in (no error)"=w202) -> ("error out"=w201:errorcluster)  [unwired: 9 in, 1 out]
          }
        }
        n79 = call <vilib>:"Add State(s) to Queue__jki_lib_state_machine.vi"("State(s) in (\"\")"=w198) -> ("States Out"=w197:string)  [unwired: 14 in]
      }
      frame "UI: Front Panel State" {
        # "Argument"
        # "Set Front Panel Open or Closed\n(Usage: \"UI: Front Panel State >> Open|Close\")"
        n80 = Unbundle By Name(w205) -> ("Core.Current VI Reference"=w204:refnum<vi>)
        n81 = case shown="\"Close\"" w203 {
          tunnel: w207 -> [w213 w226]
          tunnel: [w215 w227] -> w206
          tunnel: w204 -> [w214 w224]
          frame "Open", Default {
            n82 = property class="VI"(reference=w214, error in=w213) -> (reference out=w211:refnum<vi>, error out=w212:errorcluster, "Front Panel.Open"=w210:bool)
            n83 = case shown="False" w210 {
              tunnel: [w218 w221] -> w215
              tunnel: w212 -> [w217 w221]
              tunnel: w211 -> [w216 _]
              frame False {
                n84 = invoke class="VI" method="FP.Open"(reference=w216, error in=w217, "Activate"=TRUE, "State"=T4."Standard") -> (error out=w218:errorcluster)  [unwired: 1 in, 4 out]
              }
              frame True {
              }
            }
          }
          frame "Close" {
            n85 = property class="VI"(reference=w224, error in=w226) -> (reference out=w223:refnum<vi>, error out=w225:errorcluster, "Front Panel.Open"=w222:bool)
            n86 = case shown="True" w222 {
              tunnel: [w228 w231] -> w227
              tunnel: w225 -> [w228 w230]
              tunnel: w223 -> [_ w229]
              frame False {
              }
              frame True {
                n87 = invoke class="VI" method="FP.Close"(reference=w229, error in=w230) -> (error out=w231:errorcluster)  [unwired: 1 in, 2 out]
              }
            }
          }
        }
        n88 = call <vilib>:"Add State(s) to Queue__jki_lib_state_machine.vi"("State(s) in (\"\")"=w209) -> ("States Out"=w208:string)  [unwired: 14 in]
      }
      frame "---------- Macro ----------" {
        # "Do not put any code in this frame.\n(It is a separator no-op. You can make a copy of this frame to create a new Macro frame)"
        n89 = call <vilib>:"Add State(s) to Queue__jki_lib_state_machine.vi"("State(s) in (\"\")"=w235) -> ("States Out"=w234:string)  [unwired: 14 in]
      }
      frame "Macro: Initialize" {
        w236 = "Data: Initialize\nInitialize Core Data\nUI: Initialize\nUI: Front Panel State >> Open"  # Data: Initialize Initialize Core Data UI: Initialize UI: Front Panel State >> Open
        # "Initialization Macro\n(This is called once, when the VI starts)"
        n90 = call <vilib>:"Add State(s) to Queue__jki_lib_state_machine.vi"("State(s) in Front (\"\")"=w236, "State(s) in (\"\")"=w240) -> ("States Out"=w239:string)  [unwired: 13 in]
      }
      frame "Macro: Exit" {
        # "Exit Macro\n(This is called once, when the VI exits)"
        n91 = Unbundle By Name(w247) -> ("Core.Close Panel on Exit?"=w246:bool)
        n92 = Select(t="UI: Front Panel State >> Close", s=w246, f="") -> (s? t:f=w243:string)
        n93 = call <vilib>:"Add State(s) to Queue__jki_lib_state_machine.vi"("State(s) in (\"\")"=w243, "State(s) at Back (\"\")"="Data: Cleanup\nExit") -> ("States Out"=w241:string)  [unwired: 13 in]
        n94 = call <vilib>:"Add State(s) to Queue__jki_lib_state_machine.vi"("State(s) in Front (\"\")"=w241, "State(s) in (\"\")"=w250) -> ("States Out"=w249:string)  [unwired: 13 in]
      }
      frame "---------- New Category ----------" {
        # "Template Separator\n(You can make a copy of, or modify, this frame)"
        n95 = call <vilib>:"Add State(s) to Queue__jki_lib_state_machine.vi"("State(s) in (\"\")"=w254) -> ("States Out"=w253:string)  [unwired: 14 in]
      }
      frame "Action: Group1" {
        # "Template Separator\n(You can make a copy of, or modify, this frame)"
        n96 = Multiply(x="ms exposure", y=1000000.0) -> (x*y=w259:dbl)
        n97 = property on="exposure::1" class="DigNum (strict)"(error in=w276, "Val(Sgnl)"="ms exposure") -> (error out=w275:errorcluster)  [unwired: 1 in, 1 out]
        n98 = property on="exposure::2" class="DigNum (strict)"(error in=w275, "Val(Sgnl)"="ms exposure") -> (error out=w274:errorcluster)  [unwired: 1 in, 1 out]
        n99 = property on="exposure::3" class="DigNum (strict)"(error in=w274, "Val(Sgnl)"="ms exposure") -> (error out=w273:errorcluster)  [unwired: 1 in, 1 out]
        n100 = property on="exposure::4" class="DigNum (strict)"(error in=w273, "Val(Sgnl)"="ms exposure") -> (error out=w271:errorcluster)  [unwired: 1 in, 1 out]
        n101 = property on="exposure::6" class="DigNum (strict)"(error in=w271, "Val(Sgnl)"="ms exposure") -> (error out=w270:errorcluster)  [unwired: 1 in, 1 out]
        n102 = property on="exposure::7" class="DigNum (strict)"(error in=w270, "Val(Sgnl)"="ms exposure") -> (error out=w269:errorcluster)  [unwired: 1 in, 1 out]
        n103 = property on="exposure::8" class="DigNum (strict)"(error in=w269, "Val(Sgnl)"="ms exposure") -> (error out=w268:errorcluster)  [unwired: 1 in, 1 out]
        n104 = property on="exposure::10" class="DigNum (strict)"(error in=w268, "Val(Sgnl)"="ms exposure") -> (error out=w267:errorcluster)  [unwired: 1 in, 1 out]
        n105 = property on="exposure::11" class="DigNum (strict)"(error in=w267, "Val(Sgnl)"="ms exposure") -> (error out=w266:errorcluster)  [unwired: 1 in, 1 out]
        n106 = property on="exposure::12" class="DigNum (strict)"(error in=w266, "Val(Sgnl)"="ms exposure") -> (error out=w265:errorcluster)  [unwired: 1 in, 1 out]
        n107 = property on="exposure::13" class="DigNum (strict)"(error in=w265, "Val(Sgnl)"="ms exposure") -> (error out=w264:errorcluster)  [unwired: 1 in, 1 out]
        n108 = property on="exposure::14" class="DigNum (strict)"(error in=w264, "Val(Sgnl)"="ms exposure") -> (error out=w263:errorcluster)  [unwired: 1 in, 1 out]
        n109 = property on="exposure::15" class="DigNum (strict)"(error in=w263, "Val(Sgnl)"="ms exposure") -> (error out=w262:errorcluster)  [unwired: 1 in, 1 out]
        n110 = property on="exposure::16" class="DigNum (strict)"(error in=w262, "Val(Sgnl)"="ms exposure") -> (error out=w260:errorcluster)  [unwired: 1 in, 1 out]
        n111 = property on="exposure::17" class="DigNum (strict)"(error in=w260, "Val(Sgnl)"="ms exposure") -> (error out=w258:errorcluster)  [unwired: 1 in, 1 out]
        n112 = property on="exposure::5" class="DigNum (strict)"(error in=w258, "Val(Sgnl)"=w259) -> (error out=w257:errorcluster)  [unwired: 1 in, 1 out]
        n113 = property on="exposure::9" class="DigNum (strict)"(error in=w257, "Val(Sgnl)"=w259) -> (error out=w256:errorcluster)  [unwired: 1 in, 1 out]
        n114 = property on="exposure::18" class="DigNum (strict)"(error in=w256, "Val(Sgnl)"=w259) -> (error out=w255:errorcluster)  [unwired: 1 in, 1 out]
        n115 = call <vilib>:"Add State(s) to Queue__jki_lib_state_machine.vi"("State(s) in (\"\")"=w279) -> ("States Out"=w278:string)  [unwired: 14 in]
      }
      frame "Action: Group2" {
        # "Template Separator\n(You can make a copy of, or modify, this frame)"
        n116 = property on="exposure::1" class="DigNum (strict)"(error in=w289, "Val(Sgnl)"="amp2inputAA") -> (error out=w288:errorcluster)  [unwired: 1 in, 1 out]
        n117 = property on="exposure::2" class="DigNum (strict)"(error in=w288, "Val(Sgnl)"="amp3inputAA") -> (error out=w287:errorcluster)  [unwired: 1 in, 1 out]
        n118 = property on="exposure::3" class="DigNum (strict)"(error in=w287, "Val(Sgnl)"="amp4inputAA") -> (error out=w286:errorcluster)  [unwired: 1 in, 1 out]
        n119 = property on="exposure::4" class="DigNum (strict)"(error in=w286, "Val(Sgnl)"="amp4outputAA") -> (error out=w285:errorcluster)  [unwired: 1 in, 1 out]
        n120 = disable-structure shown="Disabled" {
          disable-tunnel: w285 -> [_ w293]
          disable-tunnel: [_ w293] -> w283
          frame Disabled {
          }
          frame Enabled {
          }
        }
        n121 = call <vilib>:"Add State(s) to Queue__jki_lib_state_machine.vi"("State(s) in (\"\")"=w292) -> ("States Out"=w291:string)  [unwired: 14 in]
      }
      frame "Action: Group3" {
        w306 = 1000000.0 ("y")
        # "Template Separator\n(You can make a copy of, or modify, this frame)"
        n122 = property on="exposure::1" class="DigNum (strict)"(error in=w324, "Val(Sgnl)"="amp2inputAA 2") -> (error out=w323:errorcluster)  [unwired: 1 in, 1 out]
        n123 = property on="exposure::2" class="DigNum (strict)"(error in=w323, "Val(Sgnl)"="amp3inputAA 2") -> (error out=w322:errorcluster)  [unwired: 1 in, 1 out]
        n124 = Multiply(x="BcaveInAA 2", y=w306) -> (x*y=w315:dbl)
        n125 = property on="exposure::3" class="DigNum (strict)"(error in=w322, "Val(Sgnl)"="amp4inputAA 2") -> (error out=w321:errorcluster)  [unwired: 1 in, 1 out]
        n126 = Multiply(x="DMSurfaceAA 2", y=w306) -> (x*y=w304:dbl)
        n127 = property on="exposure::4" class="DigNum (strict)"(error in=w321, "Val(Sgnl)"="amp4outputAA 2") -> (error out=w320:errorcluster)  [unwired: 1 in, 1 out]
        n128 = Multiply(x="tubeInAA 2", y=w306) -> (x*y=w305:dbl)
        n129 = property on="exposure::6" class="DigNum (strict)"(error in=w320, "Val(Sgnl)"="BeamlineInAA 2") -> (error out=w319:errorcluster)  [unwired: 1 in, 1 out]
        n130 = property on="exposure::7" class="DigNum (strict)"(error in=w319, "Val(Sgnl)"="BeamlineOutAA 2") -> (error out=w318:errorcluster)  [unwired: 1 in, 1 out]
        n131 = property on="exposure::8" class="DigNum (strict)"(error in=w318, "Val(Sgnl)"="compInAA 2") -> (error out=w295:errorcluster)  [unwired: 1 in, 1 out]
        n132 = property on="exposure::12" class="DigNum (strict)"(error in=w295, "Val(Sgnl)"="expanderIn2AA 2") -> (error out=w294:errorcluster)  [unwired: 1 in, 1 out]
        n133 = property on="exposure::16" class="DigNum (strict)"(error in=w294, "Val(Sgnl)"="OapIn1AA 2") -> (error out=w316:errorcluster)  [unwired: 1 in, 1 out]
        n134 = property on="exposure::17" class="DigNum (strict)"(error in=w316, "Val(Sgnl)"="OapIn2AA 2") -> (error out=w314:errorcluster)  [unwired: 1 in, 1 out]
        n135 = property on="exposure::5" class="DigNum (strict)"(error in=w314, "Val(Sgnl)"=w315) -> (error out=w313:errorcluster)  [unwired: 1 in, 1 out]
        n136 = property on="exposure::9" class="DigNum (strict)"(error in=w313, "Val(Sgnl)"=w304) -> (error out=w312:errorcluster)  [unwired: 1 in, 1 out]
        n137 = property on="exposure::18" class="DigNum (strict)"(error in=w312, "Val(Sgnl)"=w305) -> (error out=w311:errorcluster)  [unwired: 1 in, 1 out]
        n138 = call <vilib>:"Add State(s) to Queue__jki_lib_state_machine.vi"("State(s) in (\"\")"=w327) -> ("States Out"=w326:string)  [unwired: 14 in]
      }
      frame "Action: Group4" {
        w338 = 1000000.0 ("y")
        # "Template Separator\n(You can make a copy of, or modify, this frame)"
        n139 = property on="exposure::6" class="DigNum (strict)"(error in=w329, "Val(Sgnl)"="BeamlineInAA") -> (error out=w330:errorcluster)  [unwired: 1 in, 1 out]
        n140 = property on="exposure::7" class="DigNum (strict)"(error in=w330, "Val(Sgnl)"="BeamlineOutAA") -> (error out=w331:errorcluster)  [unwired: 1 in, 1 out]
        n141 = Multiply(x="BcaveInAA", y=w338) -> (x*y=w333:dbl)
        n142 = property on="exposure::8" class="DigNum (strict)"(error in=w331, "Val(Sgnl)"="compInAA") -> (error out=w349:errorcluster)  [unwired: 1 in, 1 out]
        n143 = Multiply(x="DMSurfaceAA", y=w338) -> (x*y=w340:dbl)
        n144 = property on="exposure::12" class="DigNum (strict)"(error in=w349, "Val(Sgnl)"="expanderIn2AA") -> (error out=w350:errorcluster)  [unwired: 1 in, 1 out]
        n145 = Multiply(x="tubeInAA", y=w338) -> (x*y=w339:dbl)
        n146 = property on="exposure::16" class="DigNum (strict)"(error in=w350, "Val(Sgnl)"="OapIn1AA") -> (error out=w332:errorcluster)  [unwired: 1 in, 1 out]
        n147 = property on="exposure::17" class="DigNum (strict)"(error in=w332, "Val(Sgnl)"="OapIn2AA") -> (error out=w334:errorcluster)  [unwired: 1 in, 1 out]
        n148 = property on="exposure::5" class="DigNum (strict)"(error in=w334, "Val(Sgnl)"=w333) -> (error out=w335:errorcluster)  [unwired: 1 in, 1 out]
        n149 = property on="exposure::9" class="DigNum (strict)"(error in=w335, "Val(Sgnl)"=w340) -> (error out=w336:errorcluster)  [unwired: 1 in, 1 out]
        n150 = property on="exposure::18" class="DigNum (strict)"(error in=w336, "Val(Sgnl)"=w339) -> (error out=w328:errorcluster)  [unwired: 1 in, 1 out]
        n151 = call <vilib>:"Add State(s) to Queue__jki_lib_state_machine.vi"("State(s) in (\"\")"=w353) -> ("States Out"=w352:string)  [unwired: 14 in]
      }
    }
  }
